vi "GetText.vi"(8 "error in":errorcluster, 11 "System Diagnostics editor node in":refnum<class "System Diagnostics editor node.lvclass">) -> (0 "error out":errorcluster, 1 "additional text":string, 2 "text":string, 3 "System Diagnostics editor node out":refnum<class "System Diagnostics editor node.lvclass">, 4 "glyph":string)   [LabVIEW 2013, in "System Diagnostics editor node.lvclass"]
uses:
  System Diagnostics editor node.lvclass
  <vilib>/NI/Tag Bus Data Framework/Configuration Editor/PL Framework Configuration Tool.lvlib
  <vilib>/NI/Tag Bus Data Framework/Configuration Editor/Classes/Module editor node/module editor node.lvclass
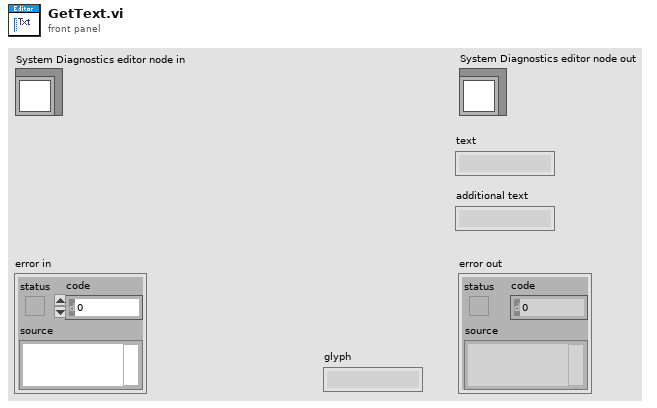
[diagram p1: front panel]
types:
  T1 = typedef "PL Framework Configuration Tool.lvlib/Glyphs Status.ctl" = enum16{"Normal", "Error", "Async"}
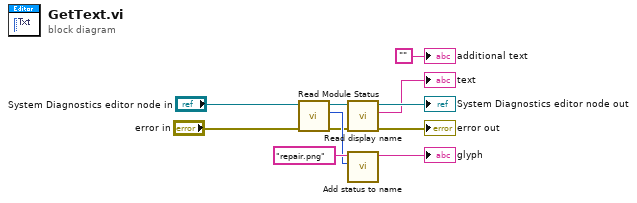
[diagram p0: block diagram]
diagram:
  n1 = call-dynamic "Read Module Status.vi"("error in"="error in", "Module Editor Node in"="System Diagnostics editor node in") -> ("error out"=w8:errorcluster, "module status"=w10:T1, "Module Editor Node out"=w9:refnum<class "System Diagnostics editor node.lvclass">)  [unwired: 7 in]
  n2 = call <vilib>:"Read display name.vi"("error in"=w8, "module editor node in"=w9) -> ("error out"=→"error out":errorcluster, "display name"=→"text":string, "module editor node out"=→"System Diagnostics editor node out":refnum<class "System Diagnostics editor node.lvclass">)  [unwired: 7 in]
  n3 = call <vilib>:"Add status to name.vi"("Status"=w10, "Name"="repair.png" ("glyph")) -> ("Name with status"=→"glyph":string)  [unwired: 9 in]
  "additional text" <- ""
